vi "locker-unlock.vi"(8 "error in (no error)":errorcluster, 11 "Queue in":refnum<queue>) -> (0 "error out":errorcluster, 3 "Queue out":refnum<queue>)   [LabVIEW 2017, in "ObjectCacherAPI.lvlib"]
uses:
  ObjectCacherAPI.lvlib
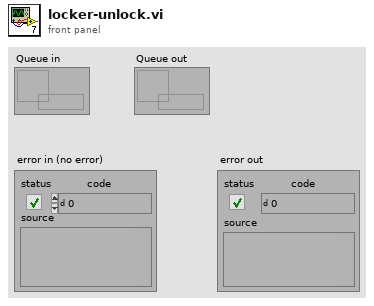
[diagram p1: front panel]
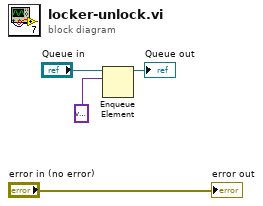
[diagram p0: block diagram]
diagram:
  n1 = Enqueue Element(queue="Queue in", element=variant) -> (queue out=→"Queue out":refnum<queue>)  [unwired: 2 in, 2 out]
  "error out" <- "error in (no error)"
